vi "GraphForm (SubVI) He.vi"() -> ()   [LabVIEW 2015]
uses:
  Global T.vi
  Global R.vi
panel:
  in  "9_ch_visible":bool=TRUE
  out "T10":dbl format="%.2f"
  in  "10_ch_visible":bool=TRUE
  in  "11_ch_visible":bool=TRUE
  in  "12_ch_visible":bool=TRUE
  in  "13_ch_visible":bool=TRUE
  in  "14_ch_visible":bool=TRUE
  in  "15_ch_visible":bool=TRUE
  in  "16_ch_visible":bool=TRUE
  in  "1_ch_v":bool=TRUE
  out "T8":dbl format="%.2f"
  out "T6":dbl format="%.2f"
  out "T2":dbl format="%.2f"
  out "T3":dbl format="%.2f"
  in  "R":T1
  in  "stop":bool
  in  "T":T2
  in  "Title":string
  out "часы":string="0"
  in  "Добавить время":dbl(ring)=300.0 items=["1 мин."=60.0, "5 мин."=300.0, "20 мин."=1200.0]
  out "мин.":string="1"
  in  "xScale +":bool
  in  "xScale -":bool
  in  "Autoscale":bool=TRUE
  in  "Т max":u16=300 min=2 max=500 step=1
  in  "Т min":u16=3 min=1 max=350
  in  "2_ch_v":bool=TRUE
  in  "3_ch_v":bool=TRUE
  in  "4_ch_v":bool=TRUE
  in  "5_ch_v":bool=TRUE
  in  "8_ch_visible":bool=TRUE
  in  "T5_col":u32(colorbox)=16711680
  in  "T3_col":u32(colorbox)=5858815
  in  "T4_col":u32(colorbox)=15688704
  in  "T1_col":u32(colorbox)=16448250
  in  "T2_col":u32(colorbox)=2132224
  out "Graphs T":dynamicdata(graph)
  # "№"
  # "T [К]"
  # "2"
  # "3"
  # "6"
  # "8"
  # "10"
  # "Интервал просмотра"
  # ":"
  # "Шкала Т"
  # "Температура, К"
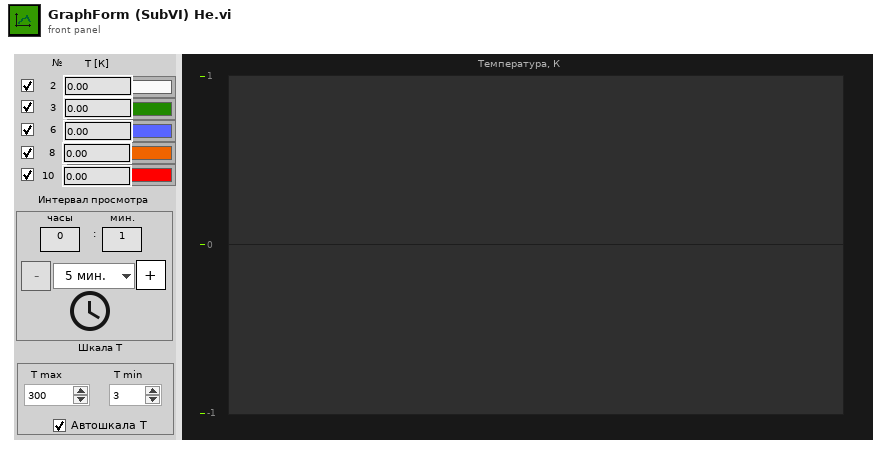
[diagram p1: front panel]
types:
  T1 = cluster{" R1":dbl, " R2":dbl, " R3":dbl, " R4":dbl, " R5":dbl, "R6":dbl, " R7":dbl, "R8":dbl, "R16":dbl, " R15":dbl, "R14":dbl, " R13":dbl, " R12":dbl, " R11":dbl, " R10":dbl, " R9":dbl}
  T2 = cluster{" T1":dbl, " T2":dbl, " T3":dbl, " T4":dbl, " T5":dbl, "T6":dbl, " T7":dbl, "T8":dbl, "T16":dbl, " T15":dbl, "T14":dbl, " T13":dbl, " T12":dbl, " T11":dbl, " T10":dbl, " T9":dbl}
  T3 = cluster{"1":dbl, " 2":dbl, " 3":dbl, "4":dbl, "5":dbl, "6":dbl, "7":dbl, "8":dbl, "9":dbl, " 10":dbl, " 11":dbl, "12":dbl, "13":dbl, "14":dbl, "15":dbl, "16":dbl}
  T4 = cluster{bool, bool, bool, bool, bool, bool, bool, bool, bool, bool, bool, bool, bool, bool, bool, bool}
  T5 = typedef "LVDateTimeRec.ctl" = cluster{"fractional second":dbl, "second":i32, "minute":i32, "hour":i32, "day of month":i32, "month":i32, "year":i32, "day of week":i32, "day of year":i32, "DST":i32}
  T6 = cluster{"1":dbl, " 2":dbl, " 3":dbl, "4":dbl, "5":dbl, "6":dbl, "7":dbl, "8":dbl, "1 2":dbl, " 10":dbl, " 11":dbl, "12":dbl, "13":dbl, "14":dbl, "15":dbl, "16":dbl}
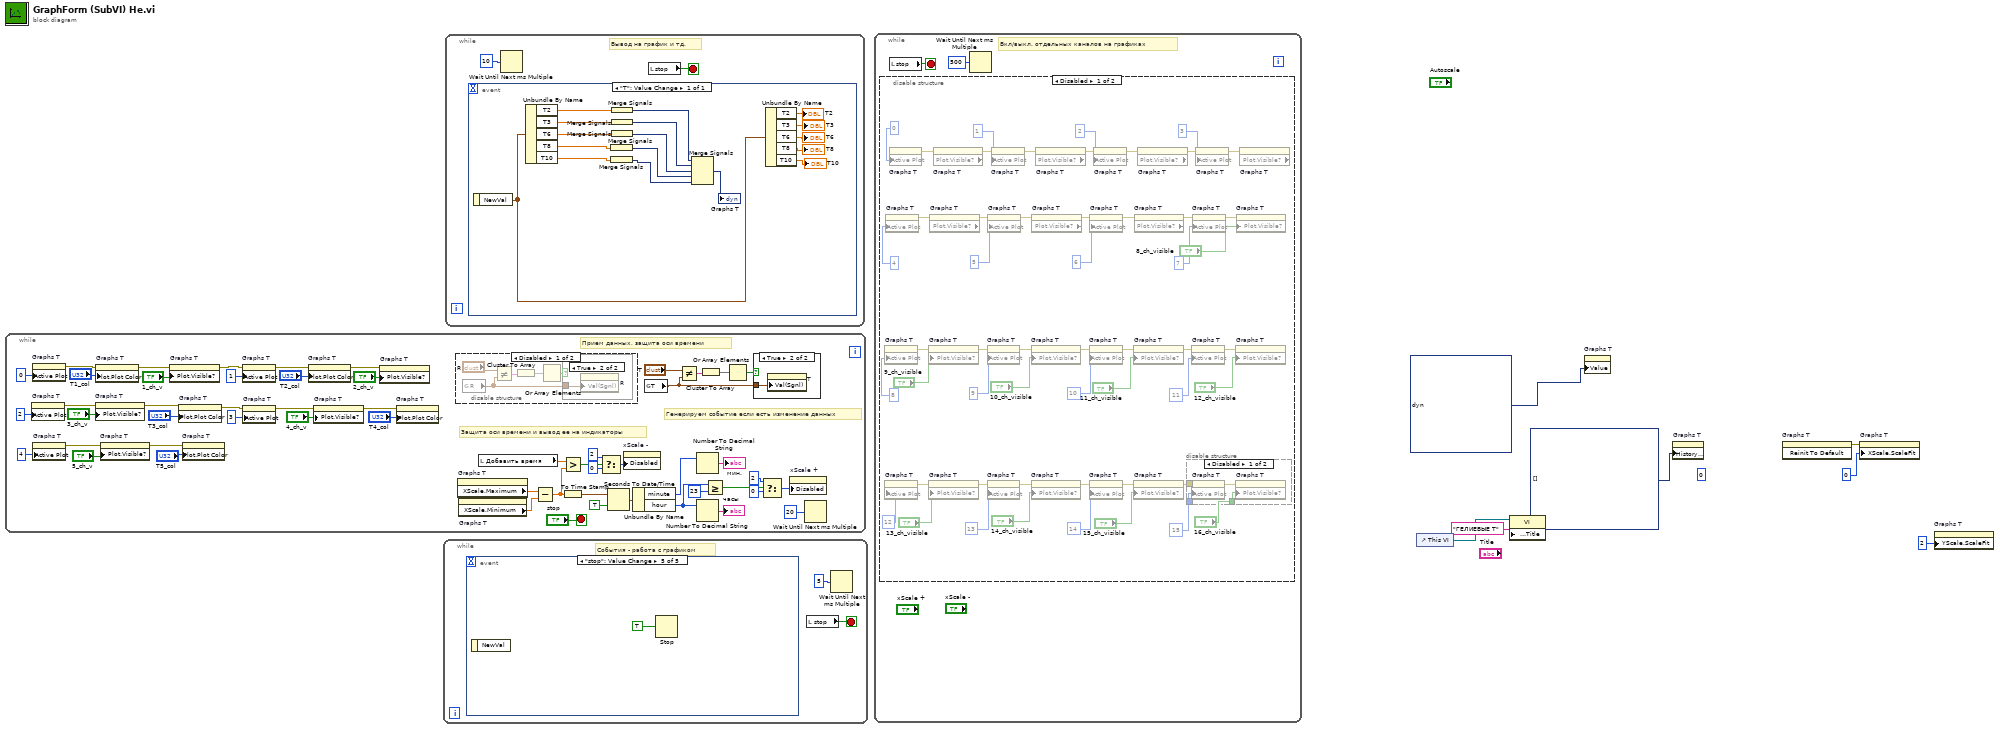
[diagram p0: block diagram]
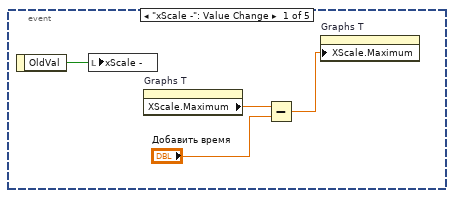
[diagram p7: hidden frame]
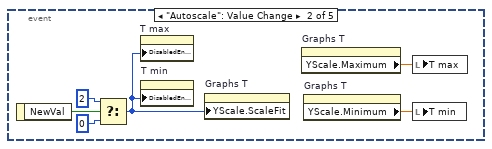
[diagram p8: hidden frame]
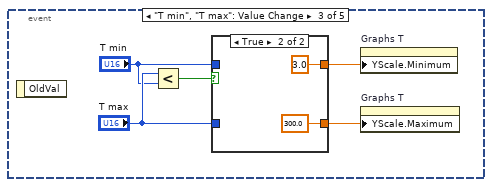
[diagram p9: hidden frame]
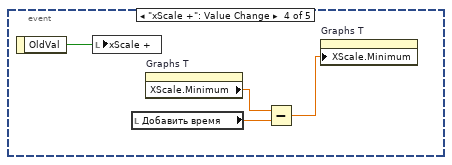
[diagram p11: hidden frame]
diagram:
  (unwired) u8 0 ("Y Scale.Scale Fit")
  n1 = while {
    stop <- "stop" stop-if-true
    # "Генерируем событие если есть изменение данных"
    # "Защита оси времени и вывод ее на индикаторы"
    # "Прием данных, защита оси времени"
    n2 = property on="Graphs T" class="WFChart (strict)"("Active Plot"=u32 2) -> (error out=w18:errorcluster)  [unwired: 2 in, 1 out]
    n3 = property on="Graphs T" class="WFChart (strict)"("Active Plot"=u32 0) -> (error out=w21:errorcluster)  [unwired: 2 in, 1 out]
    n4 = property on="Graphs T" class="WFChart (strict)"("Active Plot"=u32 4) -> (error out=w33:errorcluster)  [unwired: 2 in, 1 out]
    n5 = property on="Graphs T" class="WFChart (strict)"(error in=w18, "Plot.Visible?"="3_ch_v") -> (error out=w27:errorcluster)  [unwired: 1 in, 1 out]
    n6 = property on="Graphs T" class="WFChart (strict)"(error in=w21, "Plot.Plot Color"="T1_col") -> (error out=w22:errorcluster)  [unwired: 1 in, 1 out]
    n7 = property on="Graphs T" class="WFChart (strict)"(error in=w33, "Plot.Visible?"="5_ch_v") -> (error out=w35:errorcluster)  [unwired: 1 in, 1 out]
    n8 = property on="Graphs T" class="WFChart (strict)"(error in=w22, "Plot.Visible?"="1_ch_v") -> (error out=w13:errorcluster)  [unwired: 1 in, 1 out]
    n9 = property on="Graphs T" class="WFChart (strict)"(error in=w27, "Plot.Plot Color"="T3_col") -> (error out=w28:errorcluster)  [unwired: 1 in, 1 out]
    n10 = property on="Graphs T" class="WFChart (strict)"(error in=w35, "Plot.Plot Color"="T5_col") -> ()  [unwired: 1 in, 2 out]
    n11 = property on="Graphs T" class="WFChart (strict)"(error in=w13, "Active Plot"=u32 1) -> (error out=w24:errorcluster)  [unwired: 1 in, 1 out]
    n12 = property on="Graphs T" class="WFChart (strict)"(error in=w28, "Active Plot"=u32 3) -> (error out=w17:errorcluster)  [unwired: 1 in, 1 out]
    n13 = property on="Graphs T" class="WFChart (strict)"(error in=w24, "Plot.Plot Color"="T2_col") -> (error out=w25:errorcluster)  [unwired: 1 in, 1 out]
    n14 = property on="Graphs T" class="WFChart (strict)"(error in=w17, "Plot.Visible?"="4_ch_v") -> (error out=w29:errorcluster)  [unwired: 1 in, 1 out]
    n15 = property on="Graphs T" class="WFChart (strict)"(error in=w25, "Plot.Visible?"="2_ch_v") -> ()  [unwired: 1 in, 2 out]
    n16 = property on="Graphs T" class="WFChart (strict)"(error in=w29, "Plot.Plot Color"="T4_col") -> ()  [unwired: 1 in, 2 out]
    n17 = disable-structure shown="Disabled" {
      frame Disabled {
        n18 = global read "Global R.vi" "R"() -> (w66:T3)
        n19 = Not Equal?(x="R", y=w66) -> (x != y?=w63:T4)
        n20 = Cluster To Array(cluster=w63) -> (array=w64:bool[])
        n21 = Or Array Elements(Boolean array=w64) -> (logical OR=w65:bool)
        n22 = case shown="True" w65 {
          tunnel: w66 -> [_ w67]
          frame False {
          }
          frame True {
            n23 = property on="R" class="Clust (strict)"("Val(Sgnl)"=w67) -> ()  [unwired: 2 in, 2 out]
          }
        }
      }
      frame Enabled {
      }
    }
    n24 = property on="Graphs T" class="WFChart (strict)"() -> ("XScale.Maximum"=w61:dbl)  [unwired: 2 in, 2 out]
    n25 = property on="Graphs T" class="WFChart (strict)"() -> ("XScale.Minimum"=w60:dbl)  [unwired: 2 in, 2 out]
    n26 = local read "Добавить время"() -> (w59:dbl)
    n27 = Subtract(x=w61, y=w60) -> (x-y=w54:dbl)
    n28 = Greater?(x=w59, y=w54) -> (0:w48:bool)
    n29 = To Time Stamp(1:w54) -> (0:w57:timestamp)
    n30 = Select(t=u8 2 ("Disabled"), s=w48, f=u8 0 ("Disabled")) -> (s? t:f=w47:u8)
    n31 = Seconds To Date/Time(time stamp (now)=w57, to UTC (F)=TRUE) -> (date time rec=w56:T5)
    n32 = property on="xScale -" class="Bool (strict)"("Disabled"=w47) -> ()  [unwired: 2 in, 2 out]
    n33 = Unbundle By Name(w56) -> ("minute"=w55:i32, "hour"=w53:i32)
    n34 = global read "Global T.vi" "T"() -> (w36:T6)
    n35 = Not Equal?(x="T", y=w36) -> (x != y?=w40:T4)
    n36 = Number To Decimal String(number=w55) -> (decimal integer string=→"мин.":string)  [unwired: 1 out]
    n37 = Number To Decimal String(number=w53) -> (decimal integer string=→"часы":string)  [unwired: 1 out]
    n38 = Cluster To Array(cluster=w40) -> (array=w39:bool[])
    n39 = Greater Or Equal?(x=w53, y=23) -> (x >= y?=w43:bool)
    n40 = Or Array Elements(Boolean array=w39) -> (logical OR=w38:bool)
    n41 = case shown="True" w38 {
      tunnel: w36 -> [_ w68]
      frame False {
      }
      frame True {
        n42 = property on="T" class="Clust (strict)"("Val(Sgnl)"=w68) -> ()  [unwired: 2 in, 2 out]
      }
    }
    n43 = Select(t=u8 2 ("Disabled"), s=w43, f=u8 0 ("Disabled")) -> (s? t:f=w41:u8)
    n44 = property on="xScale +" class="Bool (strict)"("Disabled"=w41) -> ()  [unwired: 2 in, 2 out]
    n45 = Wait Until Next ms Multiple(millisecond multiple=u32 20) -> ()  [unwired: 1 out]
  }
  n46 = while {
    stop <- w69 stop-if-true
    # "События - работа с графиком"
    n47 = event shown="[4] \"stop\": Value Change" {
      selector: _ -> [_ _ _ _ _]
      dyn-events: _ -> [_ _ _ _ _]
      timeout: _ -> [_ _ _ _ _]
      event "xScale -": Value Change {
        n48 = event-data() -> ("OldVal"=w74:bool)  [unwired: 1 out]
        n49 = local write "xScale -"(w74) -> ()
        n50 = property on="Graphs T" class="WFChart (strict)"() -> ("XScale.Maximum"=w72:dbl)  [unwired: 2 in, 2 out]
        n51 = Subtract(x=w72, y="Добавить время") -> (x-y=w73:dbl)
        n52 = property on="Graphs T" class="WFChart (strict)"("XScale.Maximum"=w73) -> ()  [unwired: 2 in, 2 out]
      }
      event "Autoscale": Value Change {
        n53 = event-data() -> ("NewVal"=w75:bool)  [unwired: 1 out]
        n54 = Select(t=u8 2 ("Y Scale.Scale Fit"), s=w75, f=u8 0 ("Y Scale.Scale Fit")) -> (s? t:f=w78:u8)
        n55 = property on="Т max" class="DigNum (strict)"("DisabledEnum"=w78) -> ()  [unwired: 2 in, 2 out]
        n56 = property on="Т min" class="DigNum (strict)"("DisabledEnum"=w78) -> ()  [unwired: 2 in, 2 out]
        n57 = property on="Graphs T" class="WFChart (strict)"("YScale.ScaleFit"=w78) -> ()  [unwired: 2 in, 2 out]
        n58 = property on="Graphs T" class="WFChart (strict)"() -> ("YScale.Maximum"=w80:dbl)  [unwired: 2 in, 2 out]
        n59 = property on="Graphs T" class="WFChart (strict)"() -> ("YScale.Minimum"=w79:dbl)  [unwired: 2 in, 2 out]
        n60 = local write "Т max"(w80) -> ()
        n61 = local write "Т min"(w79) -> ()
      }
      event "Т min", "Т max": Value Change {
        n62 = event-data() -> ()  [unwired: 2 out]
        n63 = Less?(x="Т max", y="Т min") -> (x < y?=w83:bool)
        n64 = case shown="True" w83 {
          tunnel: [w86 300.0 ("x+1")] -> w85
          tunnel: [w87 3.0 ("x+1")] -> w84
          tunnel: "Т max" -> [w86 _]
          tunnel: "Т min" -> [w87 _]
          frame False {
          }
          frame True {
          }
        }
        n65 = property on="Graphs T" class="WFChart (strict)"("YScale.Minimum"=w84) -> ()  [unwired: 2 in, 2 out]
        n66 = property on="Graphs T" class="WFChart (strict)"("YScale.Maximum"=w85) -> ()  [unwired: 2 in, 2 out]
      }
      event "xScale +": Value Change {
        n67 = event-data() -> ("OldVal"=w93:bool)  [unwired: 1 out]
        n68 = local write "xScale +"(w93) -> ()
        n69 = local read "Добавить время"() -> (w90:dbl)
        n70 = property on="Graphs T" class="WFChart (strict)"() -> ("XScale.Minimum"=w91:dbl)  [unwired: 2 in, 2 out]
        n71 = Subtract(x=w91, y=w90) -> (x-y=w92:dbl)
        n72 = property on="Graphs T" class="WFChart (strict)"("XScale.Minimum"=w92) -> ()  [unwired: 2 in, 2 out]
      }
      event "stop": Value Change {
        n73 = event-data() -> ()  [unwired: 2 out]
        n74 = Stop(stop? (T)=TRUE) -> ()
      }
    }
    n75 = local read "stop"() -> (w69:bool)
    n76 = Wait Until Next ms Multiple(millisecond multiple=u32 5) -> ()  [unwired: 1 out]
  }
  n77 = while {
    stop <- w95 stop-if-true
    # "Вывод на график и тд."
    n78 = event shown="[0] \"T\": Value Change" {
      selector: _ -> [_]
      dyn-events: _ -> [_]
      timeout: _ -> [_]
      event "T": Value Change {
        n79 = event-data() -> ("NewVal"=w106:T2)  [unwired: 1 out]
        n80 = Unbundle By Name(w106) -> ("T2"=w113:dbl, "T3"=w112:dbl, "T6"=w111:dbl, "T8"=w104:dbl, "T10"=w103:dbl)
        n81 = Merge Signals(w104) -> (w102:dynamicdata)
        n82 = Merge Signals(w103) -> (w101:dynamicdata)
        n83 = Merge Signals(w113) -> (w110:dynamicdata)
        n84 = Merge Signals(w112) -> (w109:dynamicdata)
        n85 = Merge Signals(w111) -> (w108:dynamicdata)
        n86 = Merge Signals(w110, w109, w108, w102, w101) -> (→"Graphs T":dynamicdata)
        n87 = Unbundle By Name(w106) -> ("T2"=→"T2":dbl, "T3"=→"T3":dbl, "T6"=→"T6":dbl, "T8"=→"T8":dbl, "T10"=→"T10":dbl)
      }
    }
    n88 = Wait Until Next ms Multiple(millisecond multiple=u32 10) -> ()  [unwired: 1 out]
    n89 = local read "stop"() -> (w95:bool)
  }
  n90 = while {
    stop <- w114 stop-if-true
    # "Вкл/выкл. отдельных каналов на графиках"
    n91 = disable-structure shown="Disabled" {
      frame Disabled {
        n92 = property on="Graphs T" class="WFChart (strict)"("Active Plot"=u32 8) -> (error out=w134:errorcluster)  [unwired: 2 in, 1 out]
        n93 = property on="Graphs T" class="WFChart (strict)"("Active Plot"=u32 12) -> (error out=w129:errorcluster)  [unwired: 2 in, 1 out]
        n94 = property on="Graphs T" class="WFChart (strict)"("Active Plot"=u32 4) -> (error out=w170:errorcluster)  [unwired: 2 in, 1 out]
        n95 = property on="Graphs T" class="WFChart (strict)"("Active Plot"=u32 0) -> (error out=w171:errorcluster)  [unwired: 2 in, 1 out]
        n96 = property on="Graphs T" class="WFChart (strict)"(error in=w134, "Plot.Visible?"="9_ch_visible") -> (error out=w136:errorcluster)  [unwired: 1 in, 1 out]
        n97 = property on="Graphs T" class="WFChart (strict)"(error in=w129, "Plot.Visible?"="13_ch_visible") -> (error out=w127:errorcluster)  [unwired: 1 in, 1 out]
        n98 = property on="Graphs T" class="WFChart (strict)"(error in=w170) -> (error out=w168:errorcluster, "Plot.Visible?"=w151:bool)  [unwired: 1 in, 1 out]
        n99 = property on="Graphs T" class="WFChart (strict)"(error in=w171) -> (error out=w173:errorcluster, "Plot.Visible?"=w159:bool)  [unwired: 1 in, 1 out]
        n100 = property on="Graphs T" class="WFChart (strict)"(error in=w136, "Active Plot"=u32 9) -> (error out=w135:errorcluster)  [unwired: 1 in, 1 out]
        n101 = property on="Graphs T" class="WFChart (strict)"(error in=w127, "Active Plot"=u32 13) -> (error out=w128:errorcluster)  [unwired: 1 in, 1 out]
        n102 = property on="Graphs T" class="WFChart (strict)"(error in=w168, "Active Plot"=u32 5) -> (error out=w169:errorcluster)  [unwired: 1 in, 1 out]
        n103 = property on="Graphs T" class="WFChart (strict)"(error in=w173, "Active Plot"=u32 1) -> (error out=w172:errorcluster)  [unwired: 1 in, 1 out]
        n104 = property on="Graphs T" class="WFChart (strict)"(error in=w135, "Plot.Visible?"="10_ch_visible") -> (error out=w138:errorcluster)  [unwired: 1 in, 1 out]
        n105 = property on="Graphs T" class="WFChart (strict)"(error in=w128, "Plot.Visible?"="14_ch_visible") -> (error out=w125:errorcluster)  [unwired: 1 in, 1 out]
        n106 = property on="Graphs T" class="WFChart (strict)"(error in=w169) -> (error out=w166:errorcluster, "Plot.Visible?"=w149:bool)  [unwired: 1 in, 1 out]
        n107 = property on="Graphs T" class="WFChart (strict)"(error in=w172) -> (error out=w174:errorcluster, "Plot.Visible?"=w157:bool)  [unwired: 1 in, 1 out]
        n108 = property on="Graphs T" class="WFChart (strict)"(error in=w138, "Active Plot"=u32 10) -> (error out=w137:errorcluster)  [unwired: 1 in, 1 out]
        n109 = property on="Graphs T" class="WFChart (strict)"(error in=w125, "Active Plot"=u32 14) -> (error out=w126:errorcluster)  [unwired: 1 in, 1 out]
        n110 = property on="Graphs T" class="WFChart (strict)"(error in=w166, "Active Plot"=u32 6) -> (error out=w167:errorcluster)  [unwired: 1 in, 1 out]
        n111 = property on="Graphs T" class="WFChart (strict)"(error in=w174, "Active Plot"=u32 2) -> (error out=w161:errorcluster)  [unwired: 1 in, 1 out]
        n112 = property on="Graphs T" class="WFChart (strict)"(error in=w137, "Plot.Visible?"="11_ch_visible") -> (error out=w140:errorcluster)  [unwired: 1 in, 1 out]
        n113 = property on="Graphs T" class="WFChart (strict)"(error in=w126, "Plot.Visible?"="15_ch_visible") -> (error out=w124:errorcluster)  [unwired: 1 in, 1 out]
        n114 = property on="Graphs T" class="WFChart (strict)"(error in=w167) -> (error out=w164:errorcluster, "Plot.Visible?"=w147:bool)  [unwired: 1 in, 1 out]
        n115 = property on="Graphs T" class="WFChart (strict)"(error in=w161) -> (error out=w162:errorcluster, "Plot.Visible?"=w155:bool)  [unwired: 1 in, 1 out]
        n116 = disable-structure shown="Disabled" {
          disable-tunnel: w124 -> [w177 _]
          disable-tunnel: u32 15 ("Active Plot") -> [w176 _]
          disable-tunnel: "16_ch_visible" -> [w175 _]
          frame Disabled {
            n117 = property on="Graphs T" class="WFChart (strict)"(error in=w177, "Active Plot"=w176) -> (error out=w178:errorcluster)  [unwired: 1 in, 1 out]
            n118 = property on="Graphs T" class="WFChart (strict)"(error in=w178, "Plot.Visible?"=w175) -> ()  [unwired: 1 in, 2 out]
          }
          frame Enabled {
          }
        }
        n119 = property on="Graphs T" class="WFChart (strict)"(error in=w140, "Active Plot"=u32 11) -> (error out=w139:errorcluster)  [unwired: 1 in, 1 out]
        n120 = property on="Graphs T" class="WFChart (strict)"(error in=w164, "Active Plot"=u32 7) -> (error out=w165:errorcluster)  [unwired: 1 in, 1 out]
        n121 = property on="Graphs T" class="WFChart (strict)"(error in=w162, "Active Plot"=u32 3) -> (error out=w163:errorcluster)  [unwired: 1 in, 1 out]
        n122 = property on="Graphs T" class="WFChart (strict)"(error in=w139, "Plot.Visible?"="12_ch_visible") -> ()  [unwired: 1 in, 2 out]
        n123 = property on="Graphs T" class="WFChart (strict)"(error in=w165, "Plot.Visible?"="8_ch_visible") -> ()  [unwired: 1 in, 2 out]
        n124 = property on="Graphs T" class="WFChart (strict)"(error in=w163) -> ("Plot.Visible?"=w153:bool)  [unwired: 1 in, 2 out]
      }
      frame Enabled {
      }
    }
    n125 = local read "stop"() -> (w114:bool)
    n126 = Wait Until Next ms Multiple(millisecond multiple=u32 500) -> ()  [unwired: 1 out]
  }
  n127 = control-ref of="This VI"() -> (w2:refnum<vi>)
  n128 = property class="VI"(reference=w2, "Front Panel.Title"="ГЕЛИЕВЫЕ Т" ("Front Panel Window:Title")) -> ()  [unwired: 1 in, 2 out]
  n129 = property on="Graphs T" class="WFChart (strict)"("Value"=dynamicdata [{"t0"=timestamp(3465273261.7246556 s since 1904-01-01), "dt"=1.0, "Y"=[0.1931097262457384]}, {"t0"=timestamp(3465273261.7246556 s since 1904-01-01), "dt"=1.0, "Y"=[0.3594116459482981]}, {"t0"=timestamp(3465273261.7246556 s since 1904-01-01), "dt"=1.0, "Y"=[0.8898205452798131]}, {"t0"=timestamp(3465273261.7246556 s since 1904-01-01), "dt"=1.0, "Y"=[0.747699236883661]}] ("Graphs")) -> ()  [unwired: 2 in, 2 out]
  n130 = property on="Graphs T" class="WFChart (strict)"("History Data"=dynamicdata[] []) -> ()  [unwired: 2 in, 2 out]
  n131 = invoke on="Graphs T" class="WFChart (strict)" method="Reinit To Default"() -> (error out=w4:errorcluster)  [unwired: 3 in, 2 out]
  n132 = property on="Graphs T" class="WFChart (strict)"(error in=w4, "XScale.ScaleFit"=u8 0 ("Y Scale.Scale Fit")) -> ()  [unwired: 1 in, 2 out]
  n133 = property on="Graphs T" class="WFChart (strict)"("YScale.ScaleFit"=u8 2 ("Y Scale.Scale Fit")) -> ()  [unwired: 2 in, 2 out]
